vi "Read Col.vi"(8 "error in (no error)":errorcluster, 11 "Beam in":refnum<class "Beam.lvclass">) -> (0 "error out":errorcluster, 2 "Col":i32, 3 "Beam out":refnum<class "Beam.lvclass">)   [LabVIEW 2021, in "Beam.lvclass"]
uses:
  Beam.lvclass
  Beam.lvclass/Beam.ctl
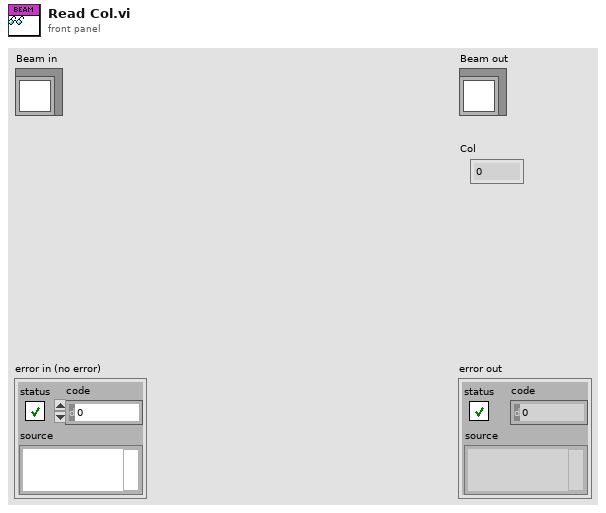
[diagram p1: front panel]
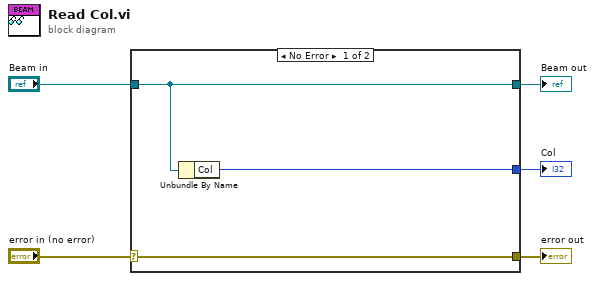
[diagram p0: block diagram]
diagram:
  n1 = case shown="No Error" "error in (no error)" {
    selector: "error in (no error)" -> [w8 w9]
    tunnel: [w8 w9] -> w4
    tunnel: [w7 w10] -> w2
    tunnel: "Beam in" -> [w7 w10]
    tunnel: [w6 _] -> w1
    frame No Error {
      n2 = Unbundle By Name(w7) -> ("Col"=w6:i32)
    }
    frame Error {
    }
  }
  "error out" <- w4
  "Beam out" <- w2
  "Col" <- w1
